vi "HW_Make_sure_stop_Acq_and_null_IO_ports.vi"(2 "error In":errorcluster, 3 "VISA Resource name IN":refnum<visa-resource-name>) -> (0 "error out":errorcluster, 1 "VISA resource name out":refnum<visa-resource-name>)   [LabVIEW 2018]
uses:
  <vilib>/Instr/_visa.llb/VISA Flush IO Buffer Mask.ctl
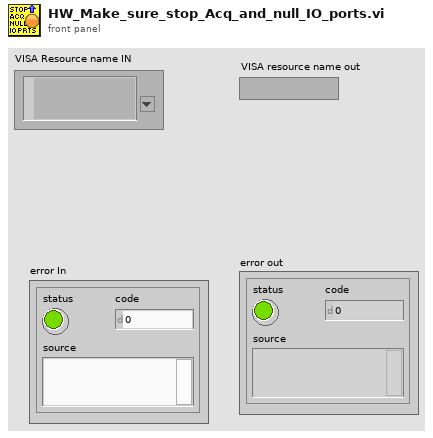
[diagram p1: front panel]
types:
  T1 = typedef "VISA Flush IO Buffer Mask.ctl" = u16
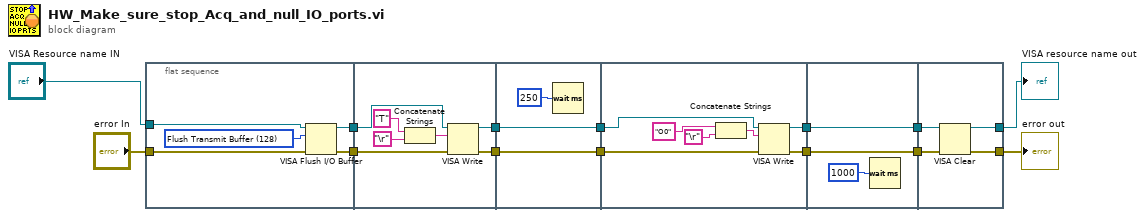
[diagram p0: block diagram]
diagram:
  n1 = flat-sequence {
    tunnel: [w16] -> w14
    tunnel: [w15] -> w13
    tunnel: "error In" -> [w17]
    tunnel: "VISA Resource name IN" -> [w19]
    tunnel: w14 -> [w26]
    tunnel: w13 -> [w25]
    tunnel: [w21] -> w12
    tunnel: [w20] -> w11
    tunnel: [w28] -> w10
    tunnel: w12 -> [w28]
    tunnel: [w27] -> w9
    tunnel: w11 -> [w27]
    tunnel: w10 -> [w33]
    tunnel: w9 -> [w32]
    tunnel: [w31] -> w8
    tunnel: [w30] -> w7
    tunnel: [w38] -> w6
    tunnel: w8 -> [w38]
    tunnel: [w37] -> w5
    tunnel: w7 -> [w37]
    tunnel: [w43] -> w3
    tunnel: w5 -> [w41]
    tunnel: w6 -> [w42]
    tunnel: [w40] -> w2
    frame #0 {
      w18 = T1 128 items=["Flush Receive Buffer"=16, "Write Transmit Buffer to Device"=32, "Flush Receive Buffer (No I/O)"=64, "Flush Transmit Buffer"=128] ("Mask")
      n2 = VISA Flush I/O Buffer(VISA resource name=w19, mask (16)=w18, error in (no error)=w17) -> (VISA resource name out=w16:refnum<visa-resource-name>, error out=w15:errorcluster)
    }
    frame #1 {
      n3 = Concatenate Strings("T" ("write buffer"), "\r") -> (w22:string)
      n4 = VISA Write(VISA resource name=w26, write buffer=w22, error in (no error)=w25) -> (VISA resource name out=w21:refnum<visa-resource-name>, error out=w20:errorcluster)  [unwired: 1 out]
    }
    frame #2 {
      n5 = Wait (ms)(milliseconds to wait=u32 250) -> ()  [unwired: 1 out]
    }
    frame #3 {
      n6 = Concatenate Strings("O0" ("write buffer"), "\r") -> (w34:string)
      n7 = VISA Write(VISA resource name=w33, write buffer=w34, error in (no error)=w32) -> (VISA resource name out=w31:refnum<visa-resource-name>, error out=w30:errorcluster)  [unwired: 1 out]
    }
    frame #4 {
      n8 = Wait (ms)(milliseconds to wait=u32 1000) -> ()  [unwired: 1 out]
    }
    frame #5 {
      n9 = VISA Clear(VISA resource name=w42, error in (no error)=w41) -> (VISA resource name out=w40:refnum<visa-resource-name>, error out=w43:errorcluster)
    }
  }
  "VISA resource name out" <- w2
  "error out" <- w3
